vi "Set Wait between Write Data (SubVI).vi"(10 "Loop Index":i32, 11 "NoResponses":i32) -> (3 "milliseconds to wait":u32)   [LabVIEW 2025]
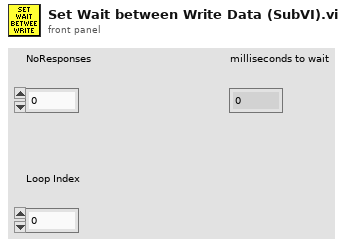
[diagram p1: front panel]
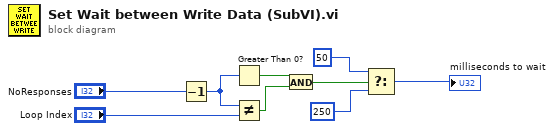
[diagram p0: block diagram]
diagram:
  n1 = Decrement(x="NoResponses") -> (x-1=w8:i32)
  n2 = Greater Than 0?(x=w8) -> (x > 0?=w6:bool)
  n3 = Not Equal?(x=w8, y="Loop Index") -> (x != y?=w7:bool)
  n4 = And(x=w6, y=w7) -> (x .and. y?=w9:bool)
  n5 = Select(t=u32 50 ("milliseconds to wait"), s=w9, f=u32 250 ("milliseconds to wait")) -> (s? t:f=→"milliseconds to wait":u32)
